vi "WinCI Get Events.vi"(8 "error in (no error)":errorcluster, 11 "source control reference in":T1) -> (0 "error out":errorcluster, 1 "filename":path, 2 "status message":string, 3 "source control reference out":T1, 4 "eventsRemaining":i32, 5 "status":i32)   [LabVIEW 2020, in "NI_SCC_WinCI.lvlib"]
uses:
  <vilib>/SourceControl/Providers/WinCI/NI_SCC_WinCI.lvlib
  <vilib>/SourceControl/sccapi/SCCAPI Refnum.ctl
  <vilib>/SourceControl/sccapi/NI_SCC.lvlib
panel:
  out "result":i32
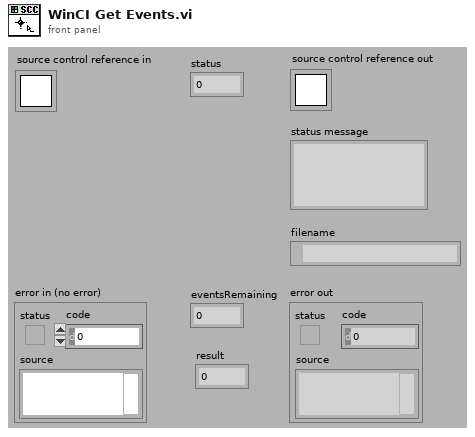
[diagram p1: front panel]
types:
  T1 = typedef "NI_SCC.lvlib/SCCAPI Refnum.ctl" = refnum<k1>
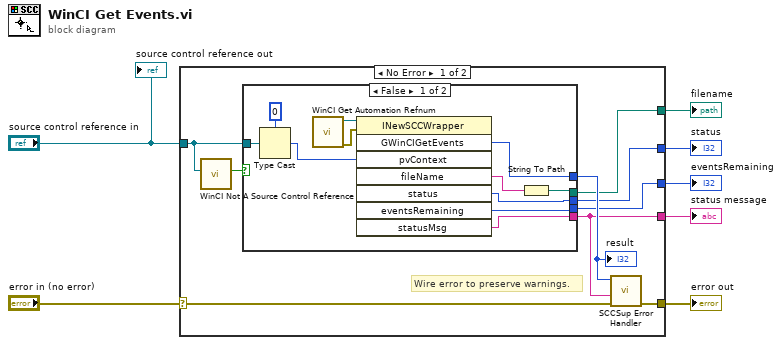
[diagram p0: block diagram]
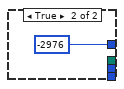
[diagram p2: hidden frame]
diagram:
  n1 = case shown="No Error" "error in (no error)" {
    selector: "error in (no error)" -> [w10 w29]
    tunnel: [w16 w29] -> w6
    tunnel: "source control reference in" -> [w8 _]
    tunnel: [w11 _] -> w4
    tunnel: [w14 _] -> w3
    tunnel: [w13 _] -> w2
    tunnel: [w12 _] -> w1
    frame No Error {
      # "Wire error to preserve warnings."
      n2 = call <vilib>:"WinCI Not A Source Control Reference.vi"("source control reference in"=w8) -> ("not a source control reference?"=w9:bool)  [unwired: 1 in, 9 out]
      n3 = case shown="False" w9 {
        tunnel: w8 -> [w27 _]
        tunnel: [w22 -2976 ("result")] -> w15
        tunnel: [w25 _] -> w14
        tunnel: [w21 _] -> w13
        tunnel: [w20 _] -> w12
        tunnel: [w19 _] -> w11
        frame False {
          n4 = Type Cast(type=u32 0, x=w27) -> (*(type *) &x=w24:u32)
          n5 = call <vilib>:"WinCI Get Automation Refnum.vi"() -> ("error out"=w18:errorcluster, "automation refnum"=w17:refnum<k7>)  [unwired: 10 out]
          n6 = invoke class="INewSCCWrapper" method="GWinCIGetEvents"(reference=w17, error in=w18, "pvContext"=w24) -> ("GWinCIGetEvents"=w22:i32, "fileName"=w23:string, "status"=w21:i32, "eventsRemaining"=w20:i32, "statusMsg"=w19:string)  [unwired: 5 in, 3 out]
          n7 = String To Path(string=w23) -> (path=w25:path)
        }
        frame True {
        }
      }
      "result" <- w15
      n8 = call <vilib>:"SCCSup Error Handler.vi"("error in (no error)"=w10, "additional message"=w11, "scc error code"=w15) -> ("error out"=w16:errorcluster)  [unwired: 1 in, 7 out]
    }
    frame Error {
    }
  }
  "error out" <- w6
  "status message" <- w4
  "filename" <- w3
  "status" <- w2
  "eventsRemaining" <- w1
  "source control reference out" <- "source control reference in"
